vi "AB_PLC_testing.vi"(6 "error in (no error)":errorcluster) -> (0 "AB plc output 10":T1, 1 "AB plc output 9":T1, 2 "AB plc output 8":T1, 3 "AB plc output 7":T1, 4 "error in (no error) 2":errorcluster)   [LabVIEW 2017]
panel:
  in  "AB plc 10":T1
  in  "AB plc 9":T1
  in  "AB plc 8":T1
  in  "AB plc 7":T1
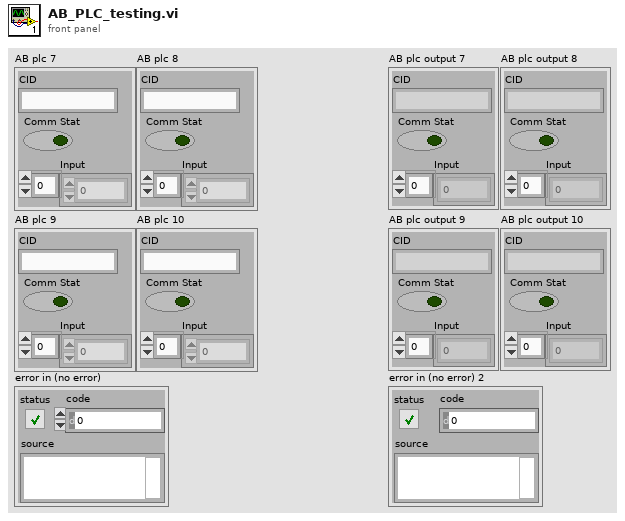
[diagram p1: front panel]
types:
  T1 = cluster{"CID":string, "Comm Stat":bool, "Input":u16[]}
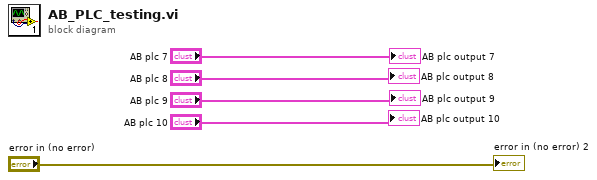
[diagram p0: block diagram]
diagram:
  "AB plc output 7" <- "AB plc 7"
  "AB plc output 8" <- "AB plc 8"
  "AB plc output 9" <- "AB plc 9"
  "AB plc output 10" <- "AB plc 10"
  "error in (no error) 2" <- "error in (no error)"
